vi "Score.vi"() -> ()   [LabVIEW 2018]
panel:
  out "Score":i32
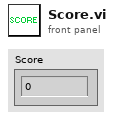
[diagram p1: front panel]
diagram:
